vi "Test_coordinate_transform.vi"() -> ()   [LabVIEW 2019]
panel:
  out "Transform":T1
  out "New Y":dbl
  out "New X":dbl
  in  "Y axis coordinate in":dbl
  in  "X axis coordinate in":dbl
  in  "Target 1":dbl[](array[numeric])
  in  "Target 0":dbl[](array[numeric])
  in  "Ref 1":dbl[](array[numeric])
  in  "Ref 0":dbl[](array[numeric])
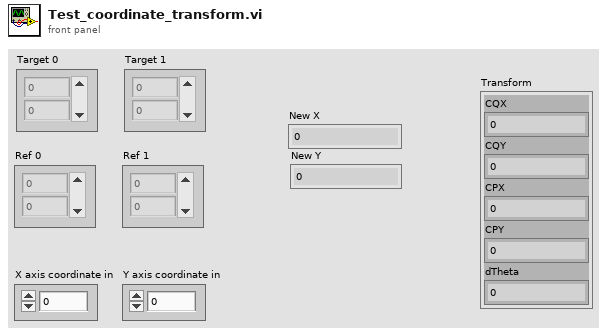
[diagram p1: front panel]
types:
  T1 = cluster{"CQX":dbl, "CQY":dbl, "CPX":dbl, "CPY":dbl, "dTheta":dbl}
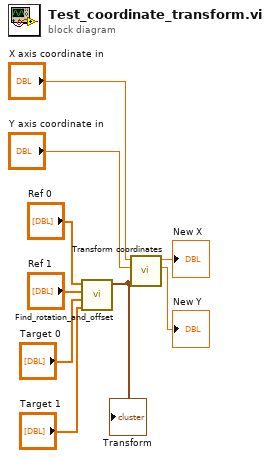
[diagram p0: block diagram]
diagram:
  n1 = call "Find_rotation_and_offset.vi"("Target 1"="Target 1", "Target 0"="Target 0", "Ref 1"="Ref 1", "Ref 0"="Ref 0") -> ("Transform"=w5:T1)  [unwired: 7 in]
  "Transform" <- w5
  n2 = call "Transform coordinates.vi"("Transform"=w5, "Y axis coordinate in"="Y axis coordinate in", "X axis coordinate in"="X axis coordinate in") -> ("New Y"=→"New Y":dbl, "New X"=→"New X":dbl)  [unwired: 7 in]
